vi "file.CreateFolder.vi"(6 "mode":T1, 8 "error in":errorcluster, 11 "DVR":T3) -> (0 "error out":errorcluster, 2 "path":T2)   [LabVIEW 2020]
uses:
  _controls/path.ctl
  _controls/data.ref.ctl
  _controls/state.ctl
  _controls/data.vars.ctl
  _controls/data.ctl
  _controls/flip.ctl
  <vilib>/vision/Image Controls.llb/IMAQ Image.ctl
  _controls/mode.ctl
  camera/camera.lvclass
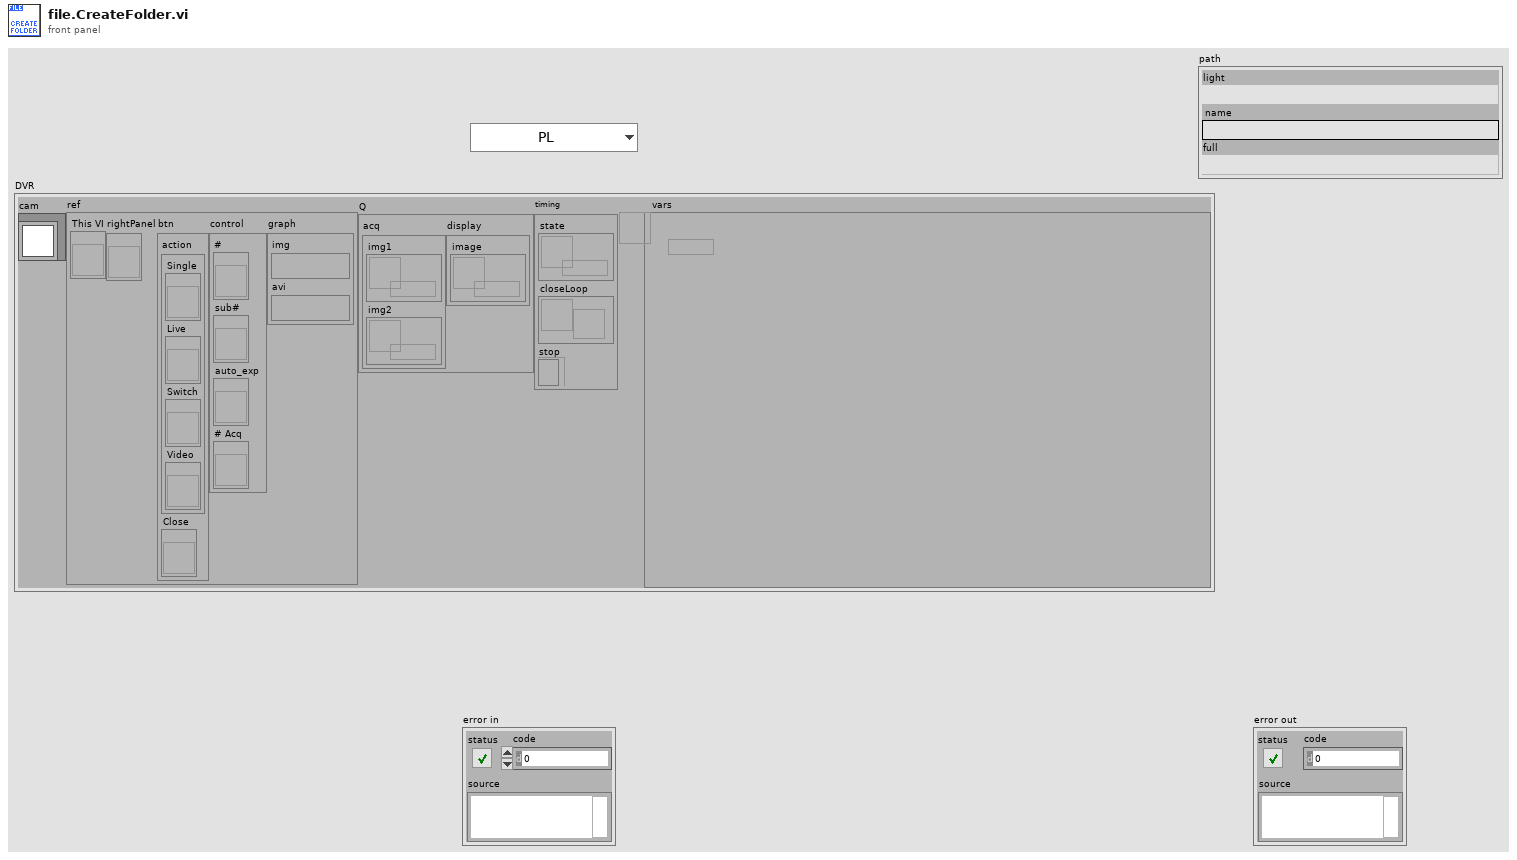
[diagram p1: front panel]
types:
  T1 = typedef "mode.ctl" = enum16{"PL", "EL"}
  T2 = typedef "path.ctl" = cluster{"light":path, "name":string, "full":path}
  T3 = typedef "data.ctl" = cluster{"cam":refnum<class "camera.lvclass">, "ref":T4, "Q":cluster{"acq":cluster{"img1":refnum<queue>, "img2":refnum<queue>}, "display":cluster{"image":refnum<queue>}}, "timing":cluster{"state":refnum<queue>, "closeLoop":refnum<notifier>, "stop":refnum<k4>}, "vars":refnum<data-value>}
  T4 = typedef "data.ref.ctl" = cluster{"This VI":refnum<vi>, "rightPanel":refnum<vi>, "btn":cluster{"action":cluster{"Single":refnum<vi>, "Live":refnum<vi>, "Switch":refnum<vi>, "Video":refnum<vi>}, "Close":refnum<vi>}, "control":cluster{"#":refnum<vi>, "sub#":refnum<vi>, "auto_exp":refnum<vi>, "# Acq":refnum<vi>}, "graph":cluster{"img":T5, "avi":T5}}
  T5 = typedef "IMAQ Image.ctl" = refnum<image>
  T6 = typedef "data.vars.ctl" = cluster{"save":cluster{"base_folder":cluster{"Folder":path, "tif":bool, "jpg":bool}, "module":string, "#":u32, "sub#":u8, "save.op":enum16{"Full", "Light"}, "same?":bool, "Shift":enum16{"Single", "Leapfrog"}, "jpg?":bool, "flip":T7}, "acq":cluster{"# Acq":u16, "rotate":bool, "FPS":dbl}, "calib.manual":cluster{"BG":cluster{"Image":u16[][], "enabled?":bool}, "FF":cluster{"Image":u16[][], "enabled?":bool}}}
  T7 = typedef "flip.ctl" = cluster{"x":bool, "y":bool}
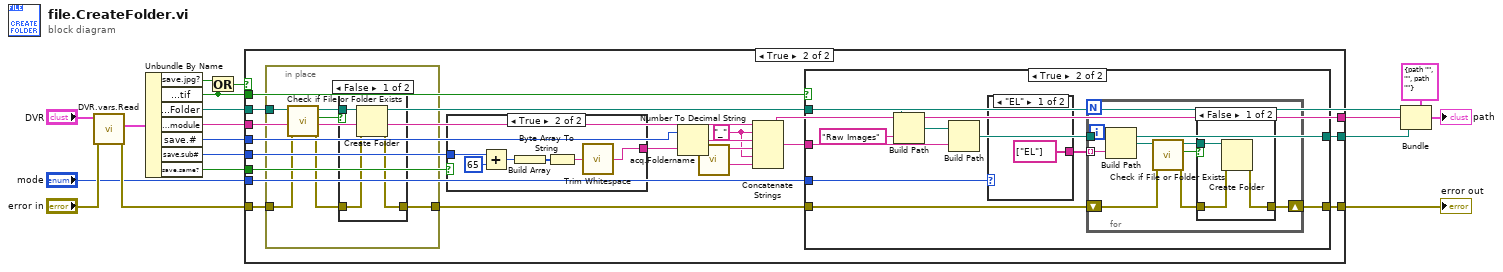
[diagram p0: block diagram]
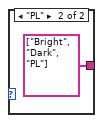
[diagram p4: hidden frame]
diagram:
  n1 = call "DVR.vars.Read.vi"("error in"="error in", "DVR.state"="DVR") -> ("error out"=w10:errorcluster, "vars"=w15:T6)  [unwired: 8 in]
  n2 = Unbundle By Name(w15) -> ("save.jpg?"=w4:bool, "save.base_folder.tif"=w2:bool, "save.base_folder.Folder"=w14:path, "save.module"=w17:string, "save.#"=w13:u32, "save.sub#"=w11:u8, "save.same?"=w12:bool)
  n3 = Or(x=w4, y=w2) -> (x .or. y?=w3:bool)
  n4 = case shown="True" w3 {
    tunnel: w17 -> [_ w35]
    tunnel: w14 -> [_ w34]
    tunnel: w13 -> [_ w33]
    tunnel: w12 -> [_ w32]
    tunnel: w11 -> [_ w31]
    tunnel: w10 -> [w19 w30]
    tunnel: [w19 w29] -> w9
    tunnel: [_ w28] -> w8
    tunnel: [_ w27] -> w7
    tunnel: w2 -> [_ w21]
    tunnel: "mode" -> [_ w20]
    frame False {
    }
    frame True {
      w24 = "_" ("string")
      n5 = in-place {
        in-place-border: w34 -> [w63]
        in-place-border: w30 -> [w62]
        in-place-border: [w61] -> w22
        n6 = call <vilib>:"Check if File or Folder Exists.vi"("error in (no error)"=w62, "path"=w63) -> ("error out"=w65:errorcluster, "file or folder exists?"=w64:bool, "dup path"=w60:path)  [unwired: 7 in]
        n7 = case shown="False" w64 {
          tunnel: w65 -> [w67 w69]
          tunnel: [w68 w69] -> w61
          tunnel: w60 -> [w66 _]
          frame False {
            n8 = Create Folder(path (use dialog)=w66, error in=w67) -> (error out=w68:errorcluster)  [unwired: 1 in, 2 out]
          }
          frame True {
          }
        }
      }
      n9 = case shown="True" w32 {
        tunnel: w31 -> [_ w72]
        tunnel: [_ w70] -> w26
        frame False {
        }
        frame True {
          n10 = Add(x=w72, y=u8 65) -> (x+y=w73:u8)
          n11 = Build Array(w73) -> (w75:u8[])
          n12 = Byte Array To String(unsigned byte array=w75) -> (string=w74:string)
          n13 = call <vilib>:"Trim Whitespace.vi"("string"=w74) -> ("trimmed string"=w70:string)  [unwired: 1 in]
        }
      }
      n14 = Number To Decimal String(number=w33) -> (decimal integer string=w25:string)  [unwired: 1 in]
      n15 = call "acq.Foldername.vi"() -> ("foldernme"=w23:string)  [unwired: 11 in]
      n16 = Concatenate Strings(w35, w24, w25, w26, w24, w23) -> (w28:string)
      n17 = case shown="True" w21 {
        tunnel: w34 -> [_ w45]
        tunnel: [w36 w44] -> w29
        tunnel: w28 -> [_ w43]
        tunnel: [_ w42] -> w27
        tunnel: w22 -> [w36 w41]
        tunnel: w20 -> [_ w37]
        frame False {
        }
        frame True {
          n18 = Build Path(base path=w45, name or relative path="Raw Images" ("string")) -> (appended path=w38:path)
          n19 = Build Path(base path=w38, name or relative path=w43) -> (appended path=w42:path)
          n20 = case shown="\"EL\"" w37 {
            tunnel: [string[] ["EL"] ("name or relative path") string[] ["Bright", "Dark", "PL"] ("name or relative path")] -> w40
            frame "EL" {
            }
            frame "PL" {
            }
          }
          n21 = for {
            tunnel: w40 -> [w55] mode=indexing
            tunnel: w42 -> [w51]
            shift-right: [w49] -> w44
            shift-left: w41 -> [w50]
            n22 = Build Path(base path=w51, name or relative path=w55) -> (appended path=w54:path)
            n23 = call <vilib>:"Check if File or Folder Exists.vi"("error in (no error)"=w50, "path"=w54) -> ("error out"=w48:errorcluster, "file or folder exists?"=w52:bool, "dup path"=w53:path)  [unwired: 7 in]
            n24 = case shown="False" w52 {
              tunnel: w53 -> [w58 _]
              tunnel: [w57 w59] -> w49
              tunnel: w48 -> [w56 w59]
              frame False {
                n25 = Create Folder(path (use dialog)=w58, error in=w56) -> (error out=w57:errorcluster)  [unwired: 1 in, 2 out]
              }
              frame True {
              }
            }
          }
        }
      }
    }
  }
  "error out" <- w9
  n26 = Bundle(cluster=T2 {"light"=path "", "name"="", "full"=path ""} ("path"), "light"=w14, "name"=w8, "full"=w7) -> (→"path":T2)
